vi "Prod - Flatten string.vi"(8 "Error In":errorcluster, 11 "Prod-Data In":T2={"Queue_Producer"=refnum, "Queue_Consumer"=refnum, "To_GUI-Error_message"=refnum, "Rx-Data"=[], "Tx-Data"=[], "Console log"="", "Communication Settings"={"Tx Protocol"=enum."Not Active", "Rx Protocol"=enum."Serial", "Serial"={"Tx Port"="", "Rx Port"="", "Baud rate"=8, "Parity"=enum."Space", "Data bits"=0, "Stop bits"=0, "Flow control"=enum."None", "Tx Resource"="", "Rx Resource"=""}, "MIDI Device"={"Input uDevice ID"=0, "Output uDevice ID"=0, "hmidiout Handle"=0, "hmidiin Handle"=0}, "Bluetooth"={"Dummy"=""}, "USB"={"Dummy"=""}}, "MIDI-Messages"=[], "Queue_Session"=refnum, "To_GUI-Pre-Session"=refnum, "To_GUI-Producer"=refnum, "Tx Info"={"Datatype"=[], "Bytesize"=[], "Strings"=[], "ByteSum"=0}, "Payload"=variant, "Timout-Time[ms]"=0, "To_GUI-Session"=refnum, "CPU(ms)"=0}) -> (0 "Error Out":errorcluster, 3 "Prod-Data Out":T2={"Queue_Producer"=refnum, "Queue_Consumer"=refnum, "To_GUI-Error_message"=refnum, "Rx-Data"=[], "Tx-Data"=[], "Console log"="", "Communication Settings"={"Tx Protocol"=enum."Not Active", "Rx Protocol"=enum."Serial", "Serial"={"Tx Port"="", "Rx Port"="", "Baud rate"=8, "Parity"=enum."Space", "Data bits"=0, "Stop bits"=0, "Flow control"=enum."None", "Tx Resource"="", "Rx Resource"=""}, "MIDI Device"={"Input uDevice ID"=0, "Output uDevice ID"=0, "hmidiout Handle"=0, "hmidiin Handle"=0}, "Bluetooth"={"Dummy"=""}, "USB"={"Dummy"=""}}, "MIDI-Messages"=[], "Queue_Session"=refnum, "To_GUI-Pre-Session"=refnum, "To_GUI-Producer"=refnum, "Tx Info"={"Datatype"=[], "Bytesize"=[], "Strings"=[], "ByteSum"=0}, "Payload"=variant, "Timout-Time[ms]"=0, "To_GUI-Session"=refnum, "CPU(ms)"=0})   [LabVIEW 2019]
doc: "Description of VI"
uses:
  Controls/Producer-Data.ctl
  Common/Controls/Application_Message.ctl
  Common/Controls/Application_State.ctl
  Common/Controls/Communication_Settings.ctl
  Common/Controls/Communication_Protocols.ctl
  MIDI/Controls/MIDI-Message_Array.ctl
  MIDI/Controls/MIDI-Message_Cluster.ctl
  MIDI/Controls/Meta_Commands.ctl
  Controls/Prod - Tx_Info.ctl
  <vilib>/Utility/error.llb/DialogType.ctl
panel:
  out "Control Tab":T1(tab)
  out "Flattened String Out":string[](array[string])
  out "Error Message":string
  out "VI-filename":string
  out "VI Path":path
  out "Code Size":u32
  out "Revision Number":u32
  in  "Tool Bar:Visible":bool
  out "VI-Name":string
  # "Settings"
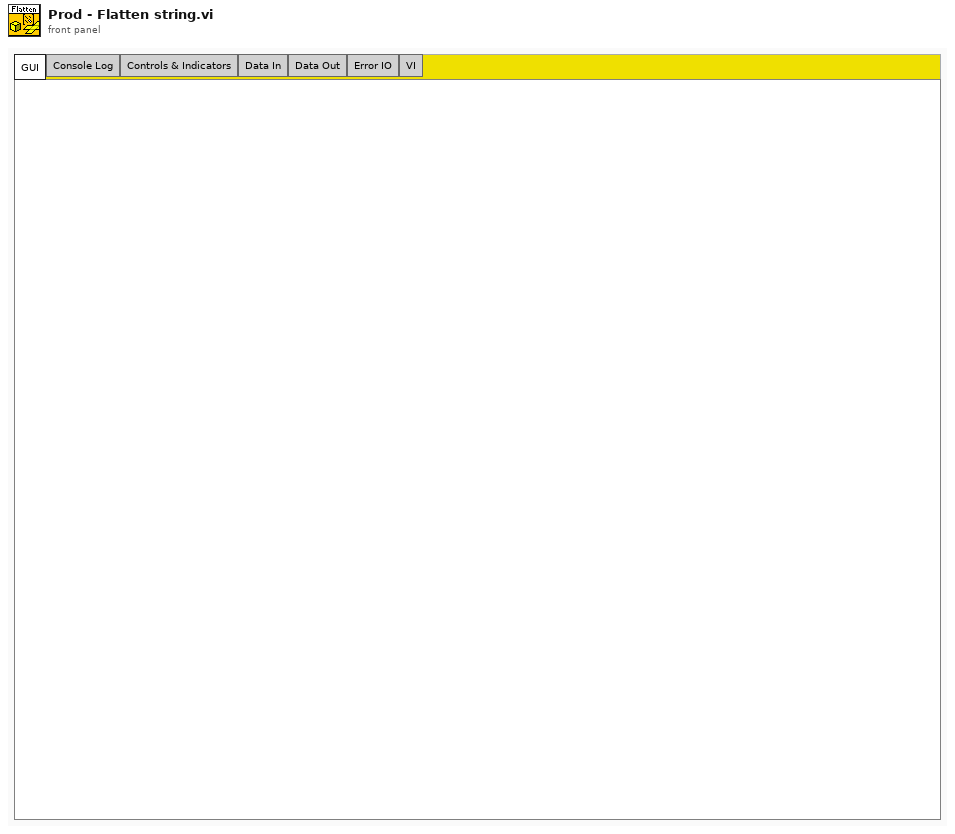
[diagram p1: front panel]
types:
  T1 = enum32{"GUI", "Console Log", "Controls & Indicators", "Data In", "Data Out", "Error IO", "VI"}
  T2 = typedef "Producer-Data.ctl" = cluster{"Queue_Producer":refnum<queue>, "Queue_Consumer":refnum<queue>, "To_GUI-Error_message":refnum<user-event>, "Rx-Data":i8[], "Tx-Data":i8[], "Console log":string, "Communication Settings":T3, "MIDI-Messages":T5, "Queue_Session":refnum<queue>, "To_GUI-Pre-Session":refnum<user-event>, "To_GUI-Producer":refnum<user-event>, "Tx Info":T8, "Payload":variant, "Timout-Time[ms]":i32, "To_GUI-Session":refnum<user-event>, "CPU(ms)":u32}
  T3 = typedef "Communication_Settings.ctl" = cluster{"Tx Protocol":T4, "Rx Protocol":T4, "Serial":cluster{"Tx Port":refnum<visa-resource-name>, "Rx Port":refnum<visa-resource-name>, "Baud rate":i32, "Parity":enum16{"None", "Odd", "Even", "Mark", "Space"}, "Data bits":i32, "Stop bits":i32, "Flow control":enum16{"None", "XON/XOFF", "RTS/CTS", "XON/XOFF & RTS/CTS", "DTR/DSR", "XON/XOFF & DTR/DSR"}, "Tx Resource":refnum<visa-resource-name>, "Rx Resource":refnum<visa-resource-name>}, "MIDI Device":cluster{"Input uDevice ID":u32, "Output uDevice ID":u32, "hmidiout Handle":i32, "hmidiin Handle":i32}, "Bluetooth":cluster{"Dummy":string}, "USB":cluster{"Dummy":string}}
  T4 = typedef "Communication_Protocols.ctl" = enum16{"Serial", "Bluetooth", "USB-MIDI", "MIDI (Audio Device)", "Not Active"}
  T5 = typedef "MIDI-Message_Array.ctl" = T6[]
  T6 = typedef "MIDI-Message_Cluster.ctl" = cluster{"Message Name":string, "Meta value":i32, "Datastring":string, "Datatype":T7}
  T7 = typedef "Meta_Commands.ctl" = enum16{"No Data", "Pause", "Loop", "Wait for Rx", "Delay", "Break", "MIDI"}
  T8 = typedef "Prod - Tx_Info.ctl" = cluster{"Datatype":T7[], "Bytesize":i32[], "Strings":string[], "ByteSum":i32}
  T9 = typedef "DialogType.ctl" = u16
  T10 = enum16{"big-endian, network order", "native, host order", "little-endian"}
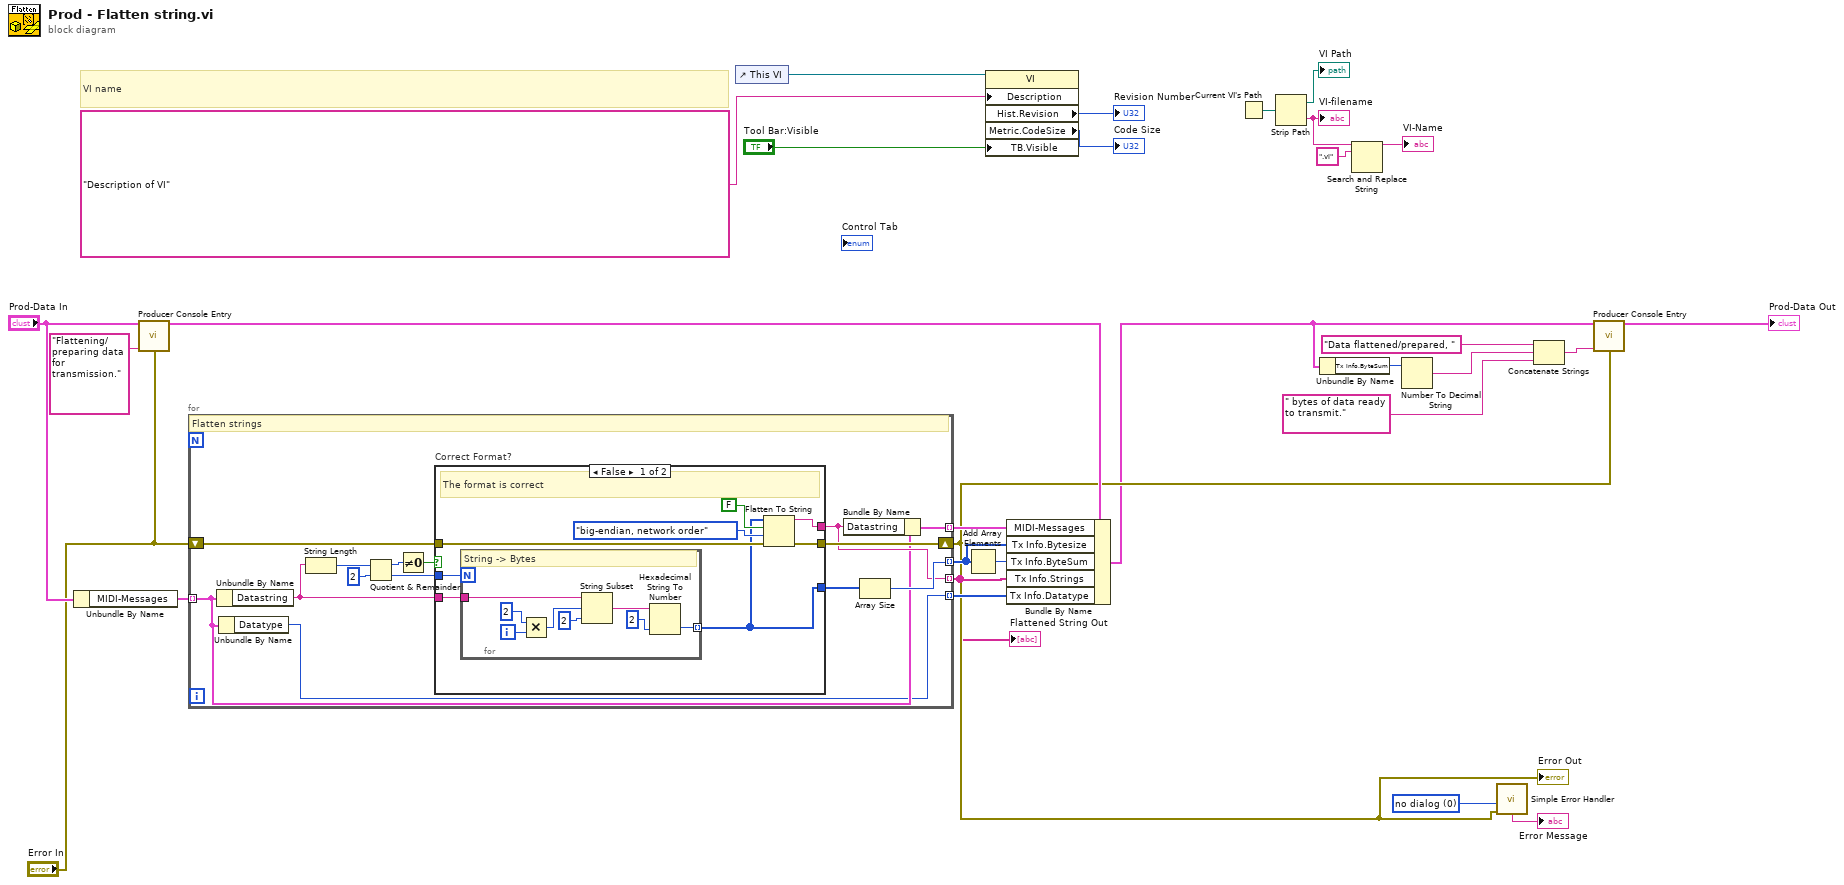
[diagram p0: block diagram]
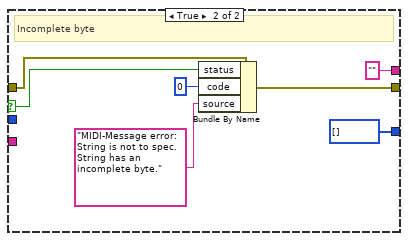
[diagram p2: hidden frame]
diagram:
  w21 = T9 0 items=["no dialog", "OK message", "continue or stop message", "OK message + warnings", "continue/stop + warnings"] ("type of dialog (OK msg:1)")
  # "VI name"
  n1 = Unbundle By Name("Prod-Data In") -> ("MIDI-Messages"=w18:T5)
  n2 = call "Producer Console Entry.vi"("Prod-Data In"="Prod-Data In", "Console Entry"="Flattening/preparing data for transmission.", "Error In"="Error In") -> ("Prod-Data Out"=w12:T2)  [unwired: 12 in]
  n3 = for {
    tunnel: w18 -> [w32] mode=indexing
    shift-right: [w37] -> w9
    shift-left: "Error In" -> [w38]
    tunnel: [w36] -> w16 mode=indexing
    tunnel: [w34] -> w1 mode=indexing
    tunnel: [w33] -> w17 mode=indexing
    tunnel: [w31] -> w14 mode=indexing
    # "Flatten strings"
    n4 = Unbundle By Name(w32) -> ("Datastring"=w41:string)
    n5 = Unbundle By Name(w32) -> ("Datatype"=w31:T7)
    n6 = String Length(string=w41) -> (length=w43:i32)
    n7 = Quotient & Remainder(x=w43, y=2) -> (x-y*floor(x/y)=w42:i32, floor(x/y)=w40:i32)
    n8 = Not Equal To 0?(x=w42) -> (x != 0?=w39:bool)
    n9 = case "Correct Format?" shown="False" w39 {
      selector: w39 -> [_ w65]
      tunnel: w41 -> [w52 _]
      tunnel: w40 -> [w51 _]
      tunnel: w38 -> [w48 w64]
      tunnel: [w47 w63] -> w37
      tunnel: [w46 "" ("data string")] -> w34
      tunnel: [w45 u8[] []] -> w35
      frame False {
        # "The format is correct"
        n10 = for {
          N: w51 -> [_]
          tunnel: w52 -> [w60]
          tunnel: [w53] -> w45 mode=indexing
          i -> [w58]
          # "String -> Bytes"
          n11 = Multiply(x=2, y=w58) -> (x*y=w56:i32)
          n12 = String Subset(string=w60, offset (0)=w56, length (rest)=i8 2 ("length (rest)")) -> (substring=w55:string)
          n13 = Hexadecimal String To Number(string=w55, default (0uL)=u8 2 ("default (0 U32)")) -> (number=w53:u8)  [unwired: 1 in, 1 out]
        }
        n14 = Flatten To String(anything=w45, prepend array or string size? (T)=FALSE, byte order (0:big-endian, network order)=T10."big-endian, network order", error in (no error)=w48) -> (data string=w46:string, error out=w47:errorcluster)  [unwired: 1 out]
      }
      frame True {
        # "Incomplete byte"
        n15 = Bundle By Name(cluster=w64, "status"=w65, "code"=0, "source"="MIDI-Message error: String is not to spec. String has an incomplete byte.") -> (w63:errorcluster)
      }
    }
    n16 = Bundle By Name(cluster=w32, "Datastring"=w34) -> (w33:T6)
    n17 = Array Size(array=w35) -> (size(s)=w36:i32)
  }
  "Error Out" <- w9
  "Flattened String Out" <- w1
  n18 = control-ref of="This VI"() -> (w27:refnum<vi>)
  n19 = Add Array Elements(numeric array=w16) -> (sum=w15:i32)
  n20 = property class="VI"(reference=w27, "Description"="Description of VI", "TB.Visible"="Tool Bar:Visible") -> ("Hist.Revision"=→"Revision Number":u32, "Metric.CodeSize"=→"Code Size":u32)  [unwired: 1 in, 2 out]
  n21 = Bundle By Name(cluster=w12, "MIDI-Messages"=w17, "Tx Info.Bytesize"=w16, "Tx Info.ByteSum"=w15, "Tx Info.Strings"=w1, "Tx Info.Datatype"=w14) -> (w7:T2)
  n22 = Current VI's Path() -> (path=w30:path)
  n23 = Strip Path(path=w30) -> (stripped path=→"VI Path":path, name=w24:string)
  "VI-filename" <- w24
  n24 = Unbundle By Name(w7) -> ("Tx Info.ByteSum"=w4:i32)
  n25 = Search and Replace String(input string=w24, search string=".vi") -> (result string=→"VI-Name":string)  [unwired: 6 in, 3 out]
  n26 = Number To Decimal String(number=w4) -> (decimal integer string=w5:string)  [unwired: 1 in]
  n27 = call <vilib>:"Simple Error Handler.vi"("type of dialog (OK msg:1)"=w21, "error in (no error)"=w9) -> ("message"=→"Error Message":string)  [unwired: 3 in, 4 out]
  n28 = Concatenate Strings("Data flattened/prepared, " ("string"), w5, " bytes of data ready to transmit." ("string")) -> (w3:string)
  n29 = call "Producer Console Entry.vi"("Prod-Data In"=w7, "Console Entry"=w3, "Error In"=w9) -> ("Prod-Data Out"=→"Prod-Data Out":T2)  [unwired: 12 in]
